vi "Speed Monitoring and Cooling System in Industrial Machinery.vi"() -> ()   [LabVIEW 2020]
uses:
  <vilib>/numeric/Random Number (Range) DBL.vi
panel:
  out "Enum":enum16{"High", "Normal", "Low", ""}(ring)
  out "FAN":string
  out "Machine Heating":bool
  out "FAN STATUS":bool
  out "RPM":dbl
  out "Temperature":string
  out "Motor Speed":dbl(knob) scale=0.0..2000.0
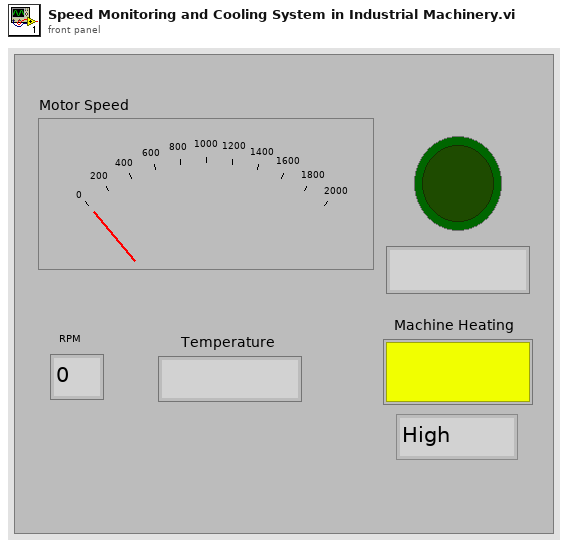
[diagram p1: front panel]
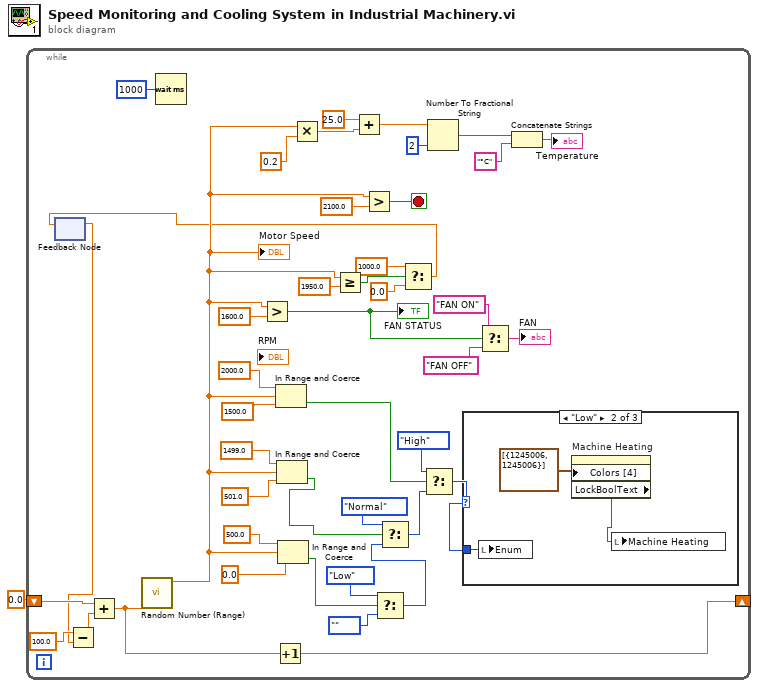
[diagram p0: block diagram]
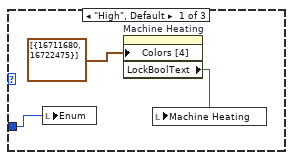
[diagram p2: hidden frame]
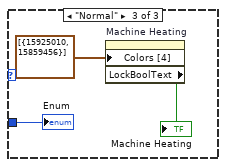
[diagram p3: hidden frame]
diagram:
  n1 = while {
    shift-right: [w22] -> _
    shift-left: 0.0 -> [w24]
    stop <- w29 stop-if-true
    n2 = feedback #1() -> (w3:dbl)  [unwired: 1 in]
    n3 = Subtract(x=100.0 ("y"), y=w3) -> (x-y=w11:dbl)
    n4 = Add(x=w24, y=w11) -> (x+y=w23:dbl)
    n5 = call-poly <vilib>:"Random Number (Range).vi"("lower bound (0)"=w23) -> ("number"=w10:dbl)  [unwired: 10 in]
    "Motor Speed" <- w10
    n6 = Wait (ms)(milliseconds to wait=u32 1000) -> ()  [unwired: 1 out]
    n7 = Greater?(x=w10, y=1600.0) -> (0:w27:bool)
    "FAN STATUS" <- w27
    n8 = Increment(x=w23) -> (x+1=w22:dbl)
    n9 = In Range and Coerce(upper limit=2000.0, x=w10, lower limit=1500.0) -> (In Range?=w21:bool)  [unwired: 1 out]
    n10 = In Range and Coerce(upper limit=1499.0, x=w10, lower limit=501.0) -> (In Range?=w15:bool)  [unwired: 1 out]
    n11 = In Range and Coerce(upper limit=500.0, x=w10, lower limit=0.0) -> (In Range?=w18:bool)  [unwired: 1 out]
    n12 = Multiply(x=w10, y=0.2) -> (x*y=w44:dbl)
    n13 = Greater Or Equal?(x=w10, y=1950.0) -> (x >= y?=w8:bool)
    n14 = Add(x=25.0, y=w44) -> (x+y=w39:dbl)
    n15 = Greater?(x=w10, y=2100.0) -> (0:w29:bool)
    n16 = Select(t=enum16{"High", "Normal", "Low", ""}."Low" ("Enum"), s=w18, f=enum16{"High", "Normal", "Low", ""}."" ("Enum")) -> (s? t:f=w16:enum16{"High", "Normal", "Low", ""})
    n17 = Select(t=enum16{"High", "Normal", "Low", ""}."Normal" ("Enum"), s=w15, f=w16) -> (s? t:f=w20:enum16{"High", "Normal", "Low", ""})
    n18 = Select(t=1000.0, s=w8, f=0.0 ("x")) -> (s? t:f=w4:dbl)
    n19 = feedback-in #1(w4) -> ()
    n20 = Select(t=enum16{"High", "Normal", "Low", ""}."High" ("Enum"), s=w21, f=w20) -> (s? t:f=w13:enum16{"High", "Normal", "Low", ""})
    n21 = Number To Fractional String(number=w39, precision (6)=i16 2) -> (F-format string=w43:string)  [unwired: 2 in]
    n22 = case shown="\"Low\"" w13 {
      tunnel: w13 -> [w48 w51 w54]
      frame "High", Default {
        n23 = local write "Enum"(w48) -> ()
        n24 = property on="Machine Heating" class="Bool (strict)"("Colors [4]"=cluster{u32, u32}[] [{16711680, 16722475}]) -> ("LockBoolText"=w46:bool)  [unwired: 2 in, 2 out]
        n25 = local write "Machine Heating"(w46) -> ()
      }
      frame "Low" {
        n26 = local write "Enum"(w51) -> ()
        n27 = property on="Machine Heating" class="Bool (strict)"("Colors [4]"=cluster{u32, u32}[] [{1245006, 1245006}]) -> ("LockBoolText"=w49:bool)  [unwired: 2 in, 2 out]
        n28 = local write "Machine Heating"(w49) -> ()
      }
      frame "Normal" {
        n29 = property on="Machine Heating" class="Bool (strict)"("Colors [4]"=cluster{u32, u32}[] [{15925010, 15859456}]) -> ("LockBoolText"=→"Machine Heating":bool)  [unwired: 2 in, 2 out]
        "Enum" <- w54
      }
    }
    n30 = Select(t="FAN ON", s=w27, f="FAN OFF") -> (s? t:f=→"FAN":string)
    n31 = Concatenate Strings(w43, "°C" ("string")) -> (→"Temperature":string)
  }
